vi "Teleop.vi"(10 "Match Info":T1={"Autonomous Elapsed Seconds"=0.0, "TeleOp Elapsed Seconds"=0.0, "Disabled Elapsed Seconds"=0.0, "Visited Autonomous"=FALSE, "Visited TeleOp"=FALSE, "Visited Disabled"=FALSE, "Autonomous Settings"={"Autonomous Style"=enum."Independent", "VI Refnum"=refnum}}, 11 "Call Context":T2) -> ()   [LabVIEW 2016]
doc: "This VI is called for each TeleOp packet received from the DS where the robot is not disabled. It is often used to read from the joysticks and update I/O or to update setpoints for timed control loops. It should complete and return within 20 milliseconds or it may miss DS packets."
uses:
  <vilib>/Rock Robotics/WPI/DriverStation/WPI_DriverStationDerivedRobotMode.ctl
  <vilib>/Rock Robotics/WPI/DriverStation/WPI_DriverStationMatch Info.ctl
  <vilib>/Rock Robotics/WPI/Utilities/WPI_GetSetVariantRefNum.vi
  <vilib>/Rock Robotics/Network Tables/NT Write Boolean Array.vi
  <vilib>/Rock Robotics/Network Tables/NT Write Numeric Array.vi
  <vilib>/Rock Robotics/Network Tables/NT Read Boolean.vi
  <vilib>/Rock Robotics/Network Tables/NT Read Number.vi
  <vilib>/Rock Robotics/WPI/Ultrasonic/WPI_SonarMB1010DigitalRefNum Registry Get.vi
  <vilib>/Rock Robotics/WPI/Ultrasonic/WPI_SonarMB1010DigitalGetRange.vi
  <vilib>/Rock Robotics/Network Tables/NT Write Number.vi
panel:
  out "current (A)":dbl
  out "number":u32
  out "Less than":bool
  out "In Range?":bool
  out "Greater":bool
  out "Distance":dbl(graph)
  in  "Auto Motor Speed":dbl=0.4 format="%#_13g"
  in  "Range":dbl format="%#_13g"
  in  "CenterPoint":dbl format="%#_13g"
  out "Distance":dbl
  out "Sample Slider 0":dbl(slide) scale=0.0..5.0
  out "Sample Boolean 1":bool
  out "Sample Boolean 0":bool
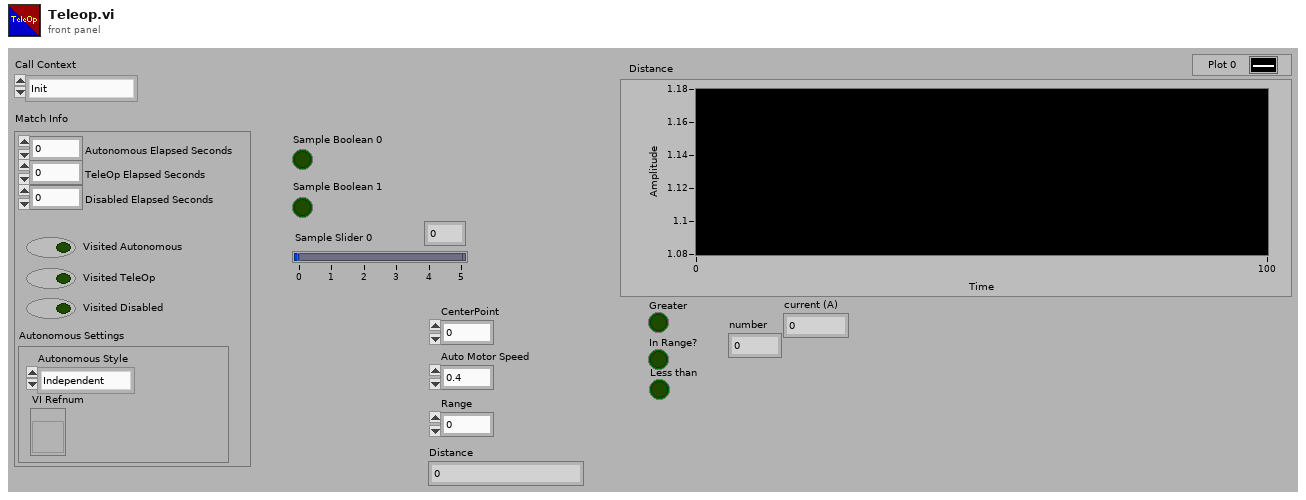
[diagram p1: front panel]
types:
  T1 = typedef "WPI_DriverStationMatch Info.ctl" = cluster{"Autonomous Elapsed Seconds":dbl, "TeleOp Elapsed Seconds":dbl, "Disabled Elapsed Seconds":dbl, "Visited Autonomous":bool, "Visited TeleOp":bool, "Visited Disabled":bool, "Autonomous Settings":cluster{"Autonomous Style":enum16{"Iterative", "Independent"}, "VI Refnum":refnum<vi>}}
  T2 = typedef "WPI_DriverStationDerivedRobotMode.ctl" = enum16{"Init", "Execute", "Stop"}
  T3 = typedef "WPI_JoystickDevRef.ctl" = cluster{"Device":T4}
  T4 = typedef "WPI_JoystickDeviceEnum.ctl" = enum16{"USB 0", "USB 1", "USB 2", "USB 3", "USB 4", "USB 5"}
  T5 = typedef "WPI_MotorControlDeviceRef.ctl" = cluster{"DeviceStatus":errorcluster, "Type":T6, "PWM":cluster{"PWM Channel":T7, "DeadBand":T8}, "CAN":cluster{"Device Number":u8, "SetOutput VI Ref":variant, "GetOutput VI Ref":variant, "Enable VI Ref":variant, "Disable VI Ref":variant, "Data":variant}, "Invert":bool}
  T6 = typedef "WPI_MotorControlType.ctl" = enum16{"PWM", "CAN"}
  T7 = typedef "FPGA_DIOPWMChannel.ctl" = enum8{"PWM 0", "PWM 1", "PWM 2", "PWM 3", "PWM 4", "PWM 5", "PWM 6", "PWM 7", "PWM 8", "PWM 9", "PWM MXP 0", "PWM MXP 1", "PWM MXP 2", "PWM MXP 3", "PWM MXP 4", "PWM MXP 5", "PWM MXP 6", "PWM MXP 7", "PWM MXP 8", "PWM MXP 9", "Invalid"}
  T8 = typedef "WPI_PWMDeadband.ctl" = cluster{"Name":string, "maxPositivePwm":i32, "minPositivePwm":i32, "centerPwm":i32, "maxNegativePwm":i32, "minNegativePwm":i32, "angularRange":u16}
  T9 = typedef "WPI_SonarMB1010DigitalDeviceRef.ctl" = cluster{"CounterDevRef":T10, "Scaling factor (s/in)":dbl}
  T10 = typedef "WPI_CounterDevRef.ctl" = cluster{"DevStatus":errorcluster, "CntIndex":T11}
  T11 = typedef "FPGA_CounterCtrSystemIndex.ctl" = enum8{"Ctr 0", "Ctr 1", "Ctr 2", "Ctr 3", "Ctr 4", "Ctr 5", "Ctr 6", "Ctr 7", "Invalid"}
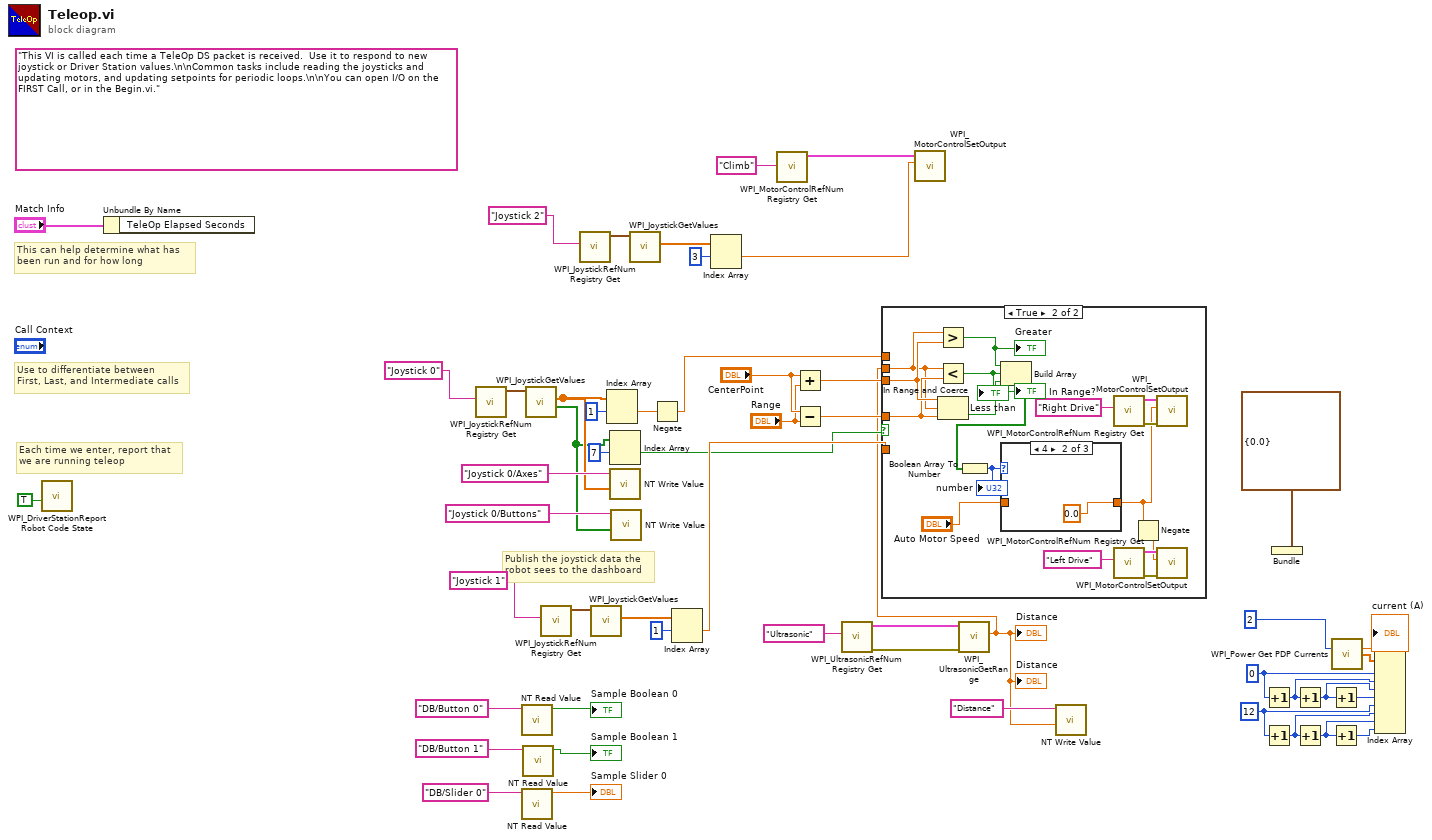
[diagram p0: block diagram]
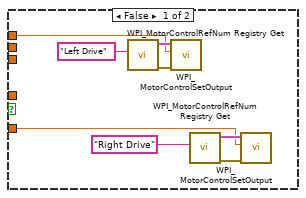
[diagram p2: hidden frame]
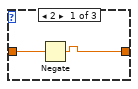
[diagram p3: hidden frame]
diagram:
  w6 = 12 ("PDP Channel")
  w10 = 0 ("PDP Channel")
  (unwired) "This VI is called each time a TeleOp DS packet is received.  Use it to respond to new joystick or Driver Station values.\n\nCommon tasks include reading the joysticks and updating motors, and updating setpoints for periodic loops.\n\nYou can open I/O on the FIRST Call, or in the Begin.vi."
  # "Publish the joystick data the\nrobot sees to the dashboard"
  # "Each time we enter, report that\nwe are running teleop"
  # "Use to differentiate between\nFirst, Last, and Intermediate calls"
  # "This can help determine what has\nbeen run and for how long"
  n1 = call <vilib>:"WPI_DriverStationReport Robot Code State.vi"("TeleOp"=TRUE ("Autonomous")) -> ()  [unwired: 10 in, 1 out]
  n2 = Unbundle By Name("Match Info") -> ()  [unwired: 1 out]
  n3 = call <vilib>:"WPI_JoystickRefNum Registry Get.vi"("refnum name"="Joystick 0") -> ("JoystickDevRef"=w50:T3)  [unwired: 1 in, 9 out]
  n4 = call-poly <vilib>:"NT Read Value.vi"("Name"="DB/Button 0" ("refnum name")) -> ("Boolean"=→"Sample Boolean 0":bool)  [unwired: 9 in, 1 out]
  n5 = call-poly <vilib>:"NT Read Value.vi"("Name"="DB/Slider 0" ("refnum name")) -> ("Numeric"=→"Sample Slider 0":dbl)  [unwired: 9 in, 1 out]
  n6 = call-poly <vilib>:"NT Read Value.vi"("Name"="DB/Button 1" ("refnum name")) -> ("Boolean"=→"Sample Boolean 1":bool)  [unwired: 9 in, 1 out]
  n7 = call <vilib>:"WPI_JoystickGetValues.vi"("JoystickDevRef"=w50) -> ("Buttons"=w20:bool[], "Axes"=w46:dbl[])  [unwired: 6 in, 3 out]
  n8 = call <vilib>:"WPI_JoystickRefNum Registry Get.vi"("refnum name"="Joystick 1") -> ("JoystickDevRef"=w38:T3)  [unwired: 1 in, 9 out]
  n9 = call <vilib>:"WPI_JoystickRefNum Registry Get.vi"("refnum name"="Joystick 2") -> ("JoystickDevRef"=w27:T3)  [unwired: 1 in, 9 out]
  n10 = call <vilib>:"WPI_JoystickGetValues.vi"("JoystickDevRef"=w38) -> ("Axes"=w39:dbl[])  [unwired: 6 in, 4 out]
  n11 = Index Array(array=w46, index #1=1 ("index")) -> (element #1=w24:dbl)  [unwired: 1 in, 1 out]
  n12 = Index Array(array=w20, index #1=7 ("index")) -> (element #1=w19:bool)  [unwired: 1 in, 1 out]
  n13 = call-poly <vilib>:"NT Write Value.vi"("Numeric Array"=w46, "Name"="Joystick 0/Axes") -> ()  [unwired: 9 in, 1 out]
  n14 = call-poly <vilib>:"NT Write Value.vi"("Boolean Array"=w20, "Name"="Joystick 0/Buttons") -> ()  [unwired: 9 in, 1 out]
  n15 = call <vilib>:"WPI_JoystickGetValues.vi"("JoystickDevRef"=w27) -> ("Axes"=w28:dbl[])  [unwired: 6 in, 4 out]
  n16 = Negate(x=w24) -> (-x=w23:dbl)
  n17 = Index Array(array=w39, index #1=1 ("index")) -> (element #1=w22:dbl)  [unwired: 1 in, 1 out]
  n18 = Index Array(array=w28, index #1=3 ("index")) -> (element #1=w25:dbl)  [unwired: 1 in, 1 out]
  n19 = call <vilib>:"WPI_MotorControlRefNum Registry Get.vi"("refnum name"="Climb") -> ("MotorControlDevRef"=w31:T5)  [unwired: 9 in, 1 out]
  n20 = Add(x="CenterPoint", y="Range") -> (x+y=w16:dbl)
  n21 = Subtract(x="CenterPoint", y="Range") -> (x-y=w15:dbl)
  n22 = call-poly <vilib>:"WPI_UltrasonicRefNum Registry Get.vi"("refnum name"="Ultrasonic") -> ("error out"=w33:errorcluster, "SonarMB1010DigitalDevRef"=w32:T9)  [unwired: 9 in]
  n23 = call <vilib>:"WPI_MotorControlSetOutput.vi"("Output"=w25, "MotorControlDevRef"=w31) -> ()  [unwired: 7 in, 3 out]
  n24 = call-poly <vilib>:"WPI_UltrasonicGetRange.vi"("error in"=w33, "SonarMB1010DigitalDevRef"=w32) -> ("Distance"=w12:dbl)  [unwired: 7 in, 2 out]
  "Distance" <- w12
  "Distance" <- w12
  n25 = case shown="True" w19 {
    tunnel: w23 -> [w53 _]
    tunnel: w22 -> [w54 _]
    tunnel: w12 -> [_ w66]
    tunnel: w16 -> [_ w69]
    tunnel: w15 -> [_ w67]
    frame False {
      n26 = call <vilib>:"WPI_MotorControlRefNum Registry Get.vi"("refnum name"="Left Drive") -> ("error out"=w55:errorcluster, "MotorControlDevRef"=w56:T5)  [unwired: 9 in]
      n27 = call <vilib>:"WPI_MotorControlSetOutput.vi"("error in (no error)"=w55, "Output"=w53, "MotorControlDevRef"=w56) -> ()  [unwired: 6 in, 3 out]
      n28 = call <vilib>:"WPI_MotorControlRefNum Registry Get.vi"("refnum name"="Right Drive") -> ("error out"=w60:errorcluster, "MotorControlDevRef"=w59:T5)  [unwired: 9 in]
      n29 = call <vilib>:"WPI_MotorControlSetOutput.vi"("error in (no error)"=w60, "Output"=w54, "MotorControlDevRef"=w59) -> ()  [unwired: 6 in, 3 out]
    }
    frame True {
      n30 = Greater?(x=w66, y=w69) -> (0:w70:bool)
      "Greater" <- w70
      n31 = Less?(x=w66, y=w67) -> (x < y?=w65:bool)
      "Less than" <- w65
      n32 = In Range and Coerce(upper limit=w69, x=w66, lower limit=w67) -> (In Range?=w68:bool)  [unwired: 1 out]
      "In Range?" <- w68
      n33 = Build Array(w70, w65, w68) -> (w64:bool[])
      n34 = Boolean Array To Number(Boolean array=w64) -> (number=w71:u32)
      "number" <- w71
      n35 = case shown="4" w71 {
        tunnel: [w78 0.0 w81] -> w62
        tunnel: "Auto Motor Speed" -> [w79 _ w81]
        frame 2 {
          n36 = Negate(x=w79) -> (-x=w78:dbl)
        }
        frame 4 {
        }
        frame 1, Default {
        }
      }
      n37 = call <vilib>:"WPI_MotorControlRefNum Registry Get.vi"("refnum name"="Right Drive") -> ("error out"=w72:errorcluster, "MotorControlDevRef"=w73:T5)  [unwired: 9 in]
      n38 = call <vilib>:"WPI_MotorControlRefNum Registry Get.vi"("refnum name"="Left Drive") -> ("error out"=w77:errorcluster, "MotorControlDevRef"=w76:T5)  [unwired: 9 in]
      n39 = Negate(x=w62) -> (-x=w61:dbl)
      n40 = call <vilib>:"WPI_MotorControlSetOutput.vi"("error in (no error)"=w72, "Output"=w62, "MotorControlDevRef"=w73) -> ()  [unwired: 6 in, 3 out]
      n41 = call <vilib>:"WPI_MotorControlSetOutput.vi"("error in (no error)"=w77, "Output"=w61, "MotorControlDevRef"=w76) -> ()  [unwired: 6 in, 3 out]
    }
  }
  n42 = call-poly <vilib>:"NT Write Value.vi"("Numeric"=w12, "Name"="Distance") -> ()  [unwired: 9 in, 1 out]
  n43 = Increment(x=w10) -> (x+1=w9:i32)
  n44 = Increment(x=w6) -> (x+1=w5:i32)
  n45 = Bundle(cluster=cluster{dbl} {0.0}) -> ()  [unwired: 1 in, 1 out]
  n46 = Increment(x=w9) -> (x+1=w7:i32)
  n47 = Increment(x=w5) -> (x+1=w3:i32)
  n48 = Increment(x=w7) -> (x+1=w8:i32)
  n49 = Increment(x=w3) -> (x+1=w4:i32)
  n50 = call <vilib>:"WPI_Power Get PDP Currents.vi"("PDP Channel"=2) -> ("current (A)"=→"current (A)":dbl, "all currents (A)"=w11:dbl[])  [unwired: 12 in, 1 out]
  n51 = Index Array(array=w11, index #1=w10, index #2=w9, index #3=w7, index #4=w8, index #5=w6, index #6=w5, index #7=w3, index #8=w4) -> ()  [unwired: 8 out]
